vi "Test Messaging.vi"() -> ()   [LabVIEW 2019, in "Instrument.Oxford1820.lvclass"]
uses:
  Instrument.Oxford1820.lvclass
  <userlib>/LevyLab/JSON-RPC/JSON-RPC.lvlib
  <userlib>/LevyLab/Instrument Framework/Instrument Types/Cryostat/Typedefs/Magnet Mode--Enum.ctl
  <userlib>/LevyLab/Instrument Framework/Instrument Types/Cryostat/Instrument.Cryostat.lvclass
  <userlib>/LevyLab/Instrument Framework/Instrument Types/Cryostat/Typedefs/Magnet Axis--Enum.ctl
  2053d202-9745-4d74-88c8-2e22be897775.vi
  Typedefs/PrivateEvents--Instrument.Oxford1820.setMagnet.ctl
panel:
  out "Field (T)":dbl[](array[numeric])
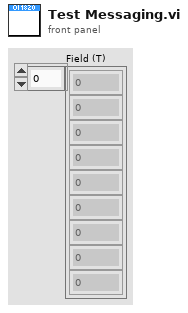
[diagram p1: front panel]
types:
  T1 = typedef "Instrument.Oxford1820.lvclass/PrivateEvents--Instrument.Oxford1820.setMagnet.ctl" = cluster{"field":dbl, "rate":dbl, "axis":T2, "mode":T3}
  T2 = typedef "Instrument.Cryostat.lvclass/Magnet Axis--Enum.ctl" = enum16{"Z", "X", "Y"}
  T3 = typedef "Instrument.Cryostat.lvclass/Magnet Mode--Enum.ctl" = enum16{"Persistent", "Driven"}
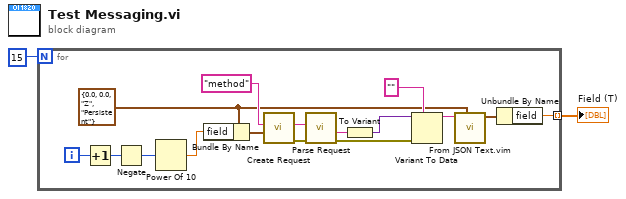
[diagram p0: block diagram]
diagram:
  n1 = for {
    N: 15 -> [_]
    tunnel: [w10] -> w2 mode=indexing
    i -> [w9]
    w3 = T1 {"field"=0.0, "rate"=0.0, "axis"=enum."Z", "mode"=enum."Persistent"} ("Set Magnet Field")
    n2 = Increment(x=w9) -> (x+1=w6:i32)
    n3 = Negate(x=w6) -> (-x=w8:i32)
    n4 = Power Of 10(x=w8) -> (10^x=w7:dbl)
    n5 = Bundle By Name(cluster=w3, "field"=w7) -> (w4:T1)
    n6 = call <userlib>:"Create Request.vi"("params"=w4, "method"="method") -> ("error out"=w14:errorcluster, "<JSON> Requests"=w18:string)  [unwired: 7 in, 1 out]
    n7 = call <userlib>:"Parse Request.vi"("error in (no error)"=w14, "<JSON> Requests"=w18) -> ("error out"=w13:errorcluster, "Params"=w17:string)  [unwired: 6 in, 2 out]
    n8 = To Variant(anything=w17) -> (Variant=w15:variant)
    n9 = Variant To Data(error in=w13, type="" ("method"), Variant=w15) -> (data=w12:string)  [unwired: 1 out]
    n10 = call "From JSON Text.vim"("Data Type and Default Value"=w3, "JSON"=w12) -> ("Data out"=w11:T1)  [unwired: 8 in, 1 out]
    n11 = Unbundle By Name(w11) -> ("field"=w10:dbl)
  }
  "Field (T)" <- w2
